vi "WaveformToCluster.vi"(8 "Target Position":dbl format="%#_13g", 9 "Start Position":dbl, 10 "Velocity":dbl, 11 "waveform":waveform(dbl)) -> (3 "output cluster":cluster{dbl[], dbl[]})   [LabVIEW 2013]
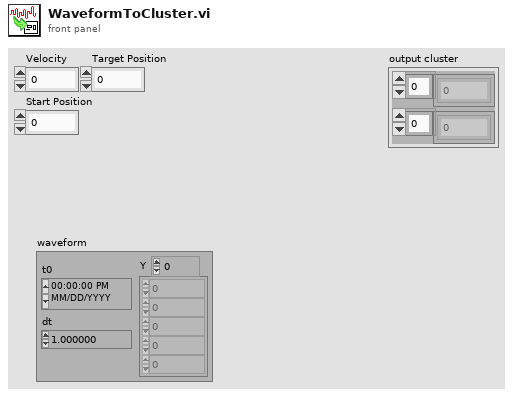
[diagram p1: front panel]
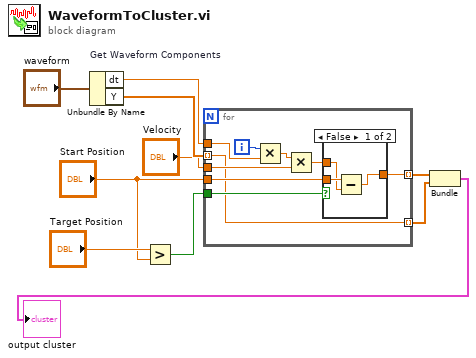
[diagram p0: block diagram]
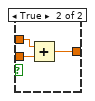
[diagram p2: hidden frame]
diagram:
  n1 = Unbundle By Name "Get Waveform Components"("waveform") -> ("dt"=w9:dbl, "Y"=w8:dbl[])
  n2 = Greater?(x="Target Position", y="Start Position") -> (0:w4:bool)
  n3 = for {
    tunnel: w9 -> [w19]
    tunnel: w8 -> [w11] mode=indexing
    tunnel: "Velocity" -> [w16]
    tunnel: "Start Position" -> [w14]
    tunnel: w4 -> [w15]
    tunnel: [w12] -> w3 mode=indexing
    tunnel: [w11] -> w2 mode=indexing
    i -> [w18]
    n4 = Multiply(x=w18, y=w19) -> (x*y=w17:dbl)
    n5 = Multiply(x=w17, y=w16) -> (x*y=w13:dbl)
    n6 = case shown="False" w15 {
      tunnel: w14 -> [w22 w25]
      tunnel: w13 -> [w21 w24]
      tunnel: [w20 w23] -> w12
      frame False {
        n7 = Subtract(x=w22, y=w21) -> (x-y=w20:dbl)
      }
      frame True {
        n8 = Add(x=w24, y=w25) -> (x+y=w23:dbl)
      }
    }
  }
  n9 = Bundle(w3, w2) -> (→"output cluster":cluster{dbl[], dbl[]})  [unwired: 1 in]
